vi "Create Templates.vi"   [LabVIEW 2014]
uses:
  <vilib>/vision/NI_Vision_Development_Module.lvlib
types:
  T1 = typedef "Image Type" = u32
  T2 = typedef "IMAQ Image.ctl" = refnum<image>
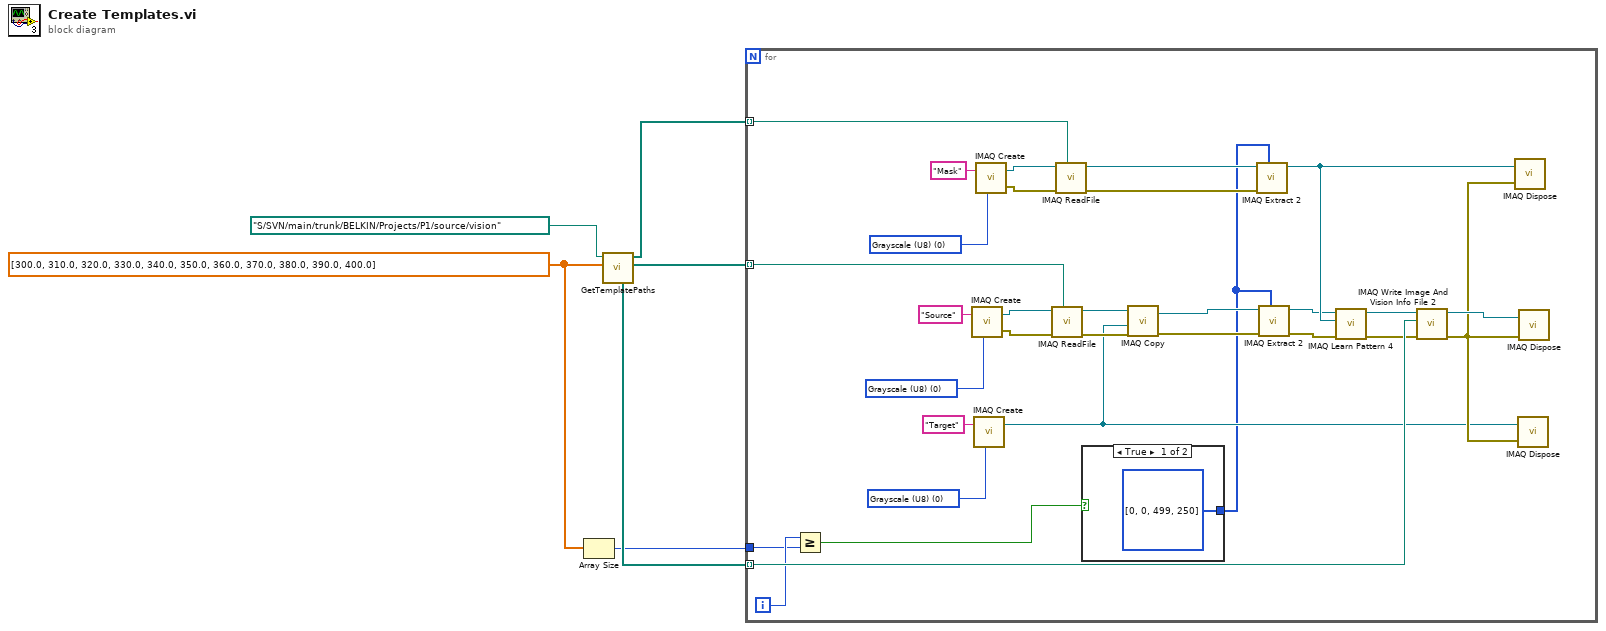
[diagram p0: block diagram]
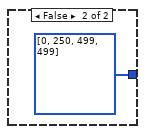
[diagram p2: hidden frame]
diagram:
  w2 = dbl[] [300.0, 310.0, 320.0, 330.0, 340.0, 350.0, 360.0, 370.0, 380.0, 390.0, 400.0]
  n1 = Array Size(array=w2) -> (size(s)=w1:i32)
  n2 = call "GetTemplatePaths.vi"("Diameters"=w2, "Folder"=path "S:/SVN/main/trunk/BELKIN/Projects/P1/source/vision" ("File Path")) -> ("TemplateSources"=w4:path[], "Masks"=w5:path[], "Templates"=w3:path[])  [unwired: 6 in, 1 out]
  n3 = for {
    tunnel: w5 -> [w33] mode=indexing
    tunnel: w4 -> [w32] mode=indexing
    tunnel: w3 -> [w23] mode=indexing
    tunnel: w1 -> [w18]
    i -> [w19]
    w27 = T1 0 items=["Grayscale (U8)", "Grayscale (I16)", "Grayscale (SGL)", "Complex (CSG)", "RGB (U32)", "HSL (U32)", "RGB (U64)", "Grayscale (U16)"] ("Image Type")
    w28 = T1 0 items=["Grayscale (U8)", "Grayscale (I16)", "Grayscale (SGL)", "Complex (CSG)", "RGB (U32)", "HSL (U32)", "RGB (U64)", "Grayscale (U16)"] ("Image Type")
    w37 = T1 0 items=["Grayscale (U8)", "Grayscale (I16)", "Grayscale (SGL)", "Complex (CSG)", "RGB (U32)", "HSL (U32)", "RGB (U64)", "Grayscale (U16)"] ("Image Type")
    n4 = Greater Or Equal?(x=w19, y=w18) -> (x >= y?=w17:bool)
    n5 = call "IMAQ Create"("Image Name"="Source", "Image Type"=w28) -> ("New Image"=w30:T2, "error out"=w31:errorcluster)  [unwired: 3 in]
    n6 = call "IMAQ Create"("Image Name"="Target", "Image Type"=w27) -> ("New Image"=w20:T2)  [unwired: 3 in, 1 out]
    n7 = call "IMAQ Create"("Image Name"="Mask", "Image Type"=w37) -> ("New Image"=w35:T2, "error out"=w34:errorcluster)  [unwired: 3 in]
    n8 = call "IMAQ ReadFile"("File Path"=w32, "error in (no error)"=w31, "Image"=w30) -> ("error out"=w24:errorcluster, "Image Out"=w25:T2)  [unwired: 4 in, 3 out]
    n9 = call "IMAQ ReadFile"("File Path"=w33, "error in (no error)"=w34, "Image"=w35) -> ("error out"=w10:errorcluster, "Image Out"=w16:T2)  [unwired: 4 in, 3 out]
    n10 = case shown="True" w17 {
      tunnel: [i32[] [0, 0, 499, 250] ("Optional Rectangle") i32[] [0, 250, 499, 499] ("Optional Rectangle")] -> w7
      frame True {
      }
      frame False {
      }
    }
    n11 = call "IMAQ Copy"("error in (no error)"=w24, "Image Dst"=w20, "Image Src"=w25) -> ("error out"=w12:errorcluster, "Image Dst Out"=w14:T2)  [unwired: 3 in]
    n12 = call "IMAQ Extract 2"("Optional Rectangle"=w7, "error in (no error)"=w10, "Image Src"=w16) -> ("Image Dst Out"=w15:T2)  [unwired: 7 in, 1 out]
    n13 = call "IMAQ Extract 2"("Optional Rectangle"=w7, "error in (no error)"=w12, "Image Src"=w14) -> ("error out"=w11:errorcluster, "Image Dst Out"=w13:T2)  [unwired: 7 in]
    n14 = call "IMAQ Learn Pattern 4"("error in (no error)"=w11, "Mask"=w15, "Image"=w13) -> ("error out"=w8:errorcluster, "Template Image Out"=w9:T2)  [unwired: 6 in, 1 out]
    n15 = call "IMAQ Write Image And Vision Info File 2"("error in (no error)"=w8, "File Path"=w23, "Image"=w9) -> ("error out"=w21:errorcluster, "Image Out (duplicate)"=w22:T2)  [unwired: 7 in]
    n16 = call "IMAQ Dispose"("Image"=w15, "error in (no error)"=w21) -> ()  [unwired: 4 in, 1 out]
    n17 = call "IMAQ Dispose"("Image"=w20, "error in (no error)"=w21) -> ()  [unwired: 4 in, 1 out]
    n18 = call "IMAQ Dispose"("Image"=w22, "error in (no error)"=w21) -> ()  [unwired: 4 in, 1 out]
  }
